vi "Get All Names and Values.vi"(8 "error in":errorcluster, 11 "Cluster in":variant) -> (0 "error out":errorcluster, 1 "Values":variant[](array[variant]), 2 "Element Names":string[](array[string]), 3 "Cluster out":variant, 4 "Cluster Name":string)   [LabVIEW 2017, in "Variant Data Manipulation.lvlib"]
doc: "Returns an array of all of the keys and an array of their corresponding values. Elements are correlated by index, so the key at a given index corresponds to the value at the same index."
uses:
  Variant Data Manipulation.lvlib
  <vilib>/Utility/Data Type/NI_Data Type.lvlib
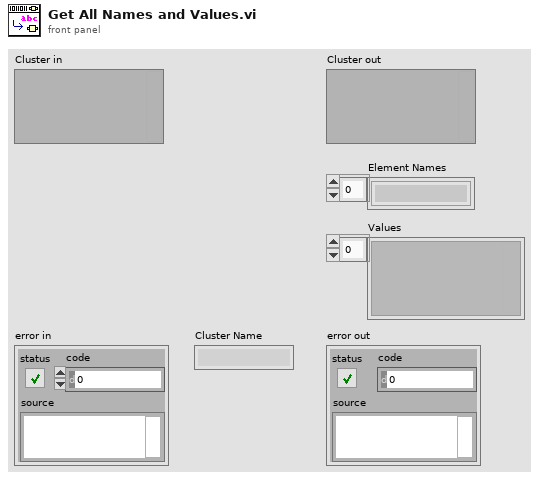
[diagram p1: front panel]
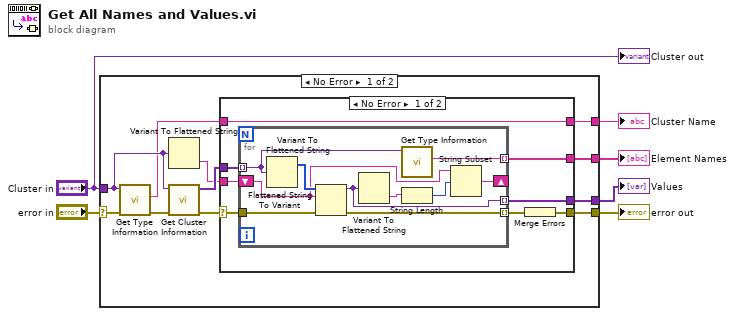
[diagram p0: block diagram]
diagram:
  n1 = case shown="No Error" "error in" {
    selector: "error in" -> [w14 w37]
    tunnel: "Cluster in" -> [w9 _]
    tunnel: [w13 w37] -> w4
    tunnel: [w12 _] -> w3
    tunnel: [w11 _] -> w2
    tunnel: [w8 _] -> w1
    frame No Error {
      n2 = call <vilib>:"Get Type Information.vi"("error in (no error)"=w14, "Variant"=w9) -> ("error out"=w10:errorcluster, "Name"=w7:string)  [unwired: 5 in, 3 out]
      n3 = Variant To Flattened String(Variant=w9) -> (data string=w15:string)  [unwired: 1 out]
      n4 = call <vilib>:"Get Cluster Information.vi"("error in (no error)"=w10, "Variant"=w9) -> ("error out"=w17:errorcluster, "Cluster Elements"=w16:variant[])  [unwired: 8 in]
      n5 = case shown="No Error" w17 {
        selector: w17 -> [w24 w36]
        tunnel: w16 -> [w23 _]
        tunnel: w15 -> [w22 _]
        tunnel: [w21 w36] -> w13
        tunnel: [w20 _] -> w12
        tunnel: [w19 _] -> w11
        tunnel: [w18 _] -> w8
        tunnel: w7 -> [w18 _]
        frame No Error {
          n6 = for {
            tunnel: w23 -> [w27] mode=indexing
            tunnel: [w34] -> w20 mode=indexing
            shift-right: [w30] -> _
            shift-left: w22 -> [w33]
            tunnel: w24 -> [w29]
            tunnel: [w28] -> w25 mode=indexing
            tunnel: [w26] -> w19 mode=indexing
            n7 = Variant To Flattened String(Variant=w27) -> (1:w35:i16[])  [unwired: 1 out]
            n8 = Flattened String To Variant(4:w29, 6:w33, 7:w35) -> (0:w28:errorcluster, 3:w34:variant)
            n9 = Variant To Flattened String(Variant=w34) -> (data string=w32:string)  [unwired: 1 out]
            n10 = call <vilib>:"Get Type Information.vi"("Variant"=w27) -> ("Name"=w26:string)  [unwired: 6 in, 4 out]
            n11 = String Length(string=w32) -> (length=w31:i32)
            n12 = String Subset(string=w33, offset (0)=w31) -> (substring=w30:string)  [unwired: 1 in]
          }
          n13 = Merge Errors(w25) -> (w21:errorcluster)
        }
        frame Error {
        }
      }
    }
    frame Error {
    }
  }
  "Element Names" <- w2
  "Values" <- w3
  "error out" <- w4
  "Cluster Name" <- w1
  "Cluster out" <- "Cluster in"
